vi "Bury.vi"(8 "Error In":errorcluster, 11 "Graves":refnum<vi>[](array[refnum])) -> (0 "Error Out":errorcluster, 3 "Change Made?":bool)   [LabVIEW 2017, in "Toolkit.lvlib"]
doc: "Burys the corpse of legacy code. This removes the grave (Diagram Disable Structure) and leaves behind the Spirit frame, which should be enabled before burying the corpse. Note, the corpse frame will no longer exists and be pernamently deleted."
uses:
  Toolkit.lvlib
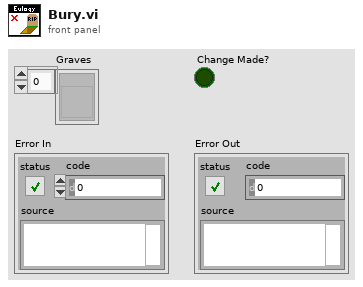
[diagram p1: front panel]
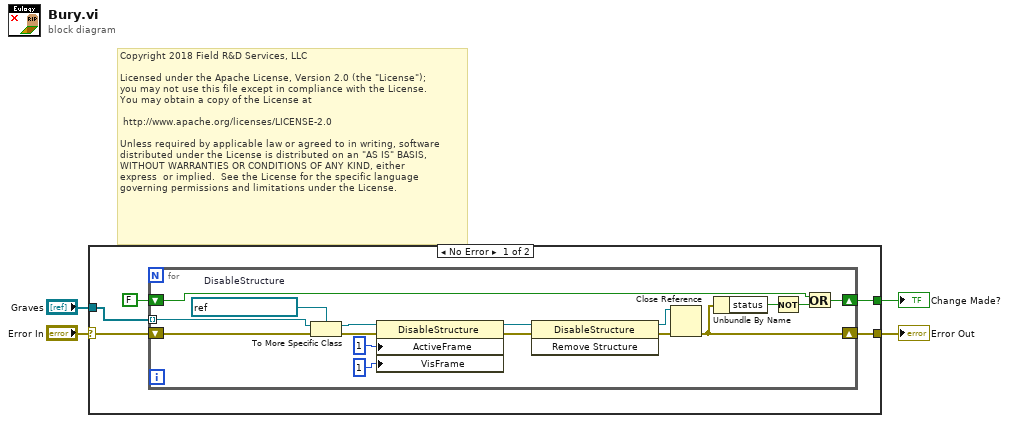
[diagram p0: block diagram]
diagram:
  # "Copyright 2018 Field R&D Services, LLC\n\nLicensed under the Apache License, Version 2.0 (the \"License\");\nyou may not use this file except in compliance with the License.\nYou may obtain a copy of the License at\n\n\thttp://www.apache.org/licenses/LICENSE-2.0\n\nUnless required by applicable law or agreed to in writing, software\ndistributed under the License is distributed on an \"AS IS\" BASIS,\nWITHOUT WARRANTIES OR CONDITIONS OF ANY KIND, either \nexpress  or implied.  See the License for the specific language \ngoverning permissions and limitations under the License."
  n1 = case shown="No Error" "Error In" {
    selector: "Error In" -> [w5 w26]
    tunnel: [w9 w26] -> w4
    tunnel: [w7 _] -> w3
    tunnel: "Graves" -> [w6 _]
    frame No Error {
      n2 = for {
        shift-right: [w12] -> w9
        shift-left: w5 -> [w20]
        tunnel: w6 -> [w21] mode=indexing
        shift-right: [w24] -> w7
        shift-left: FALSE -> [w25]
        w19 = refnum<vi> refnum  # DisableStructure
        n3 = To More Specific Class(target class=w19, reference=w21, error in=w20) -> (specific class reference=w18:refnum<vi>, error out=w17:errorcluster)
        n4 = property class="DisableStructure"(reference=w18, error in=w17, "ActiveFrame"=i16 1 ("Active Frame"), "VisFrame"=u32 1 ("Visible Frame")) -> (reference out=w15:refnum<vi>, error out=w13:errorcluster)
        n5 = invoke class="DisableStructure" method="Remove Structure"(reference=w15, error in=w13) -> (reference out=w22:refnum<vi>, error out=w23:errorcluster)  [unwired: 1 in, 1 out]
        n6 = Close Reference(reference=w22, error in (no error)=w23) -> (error out=w12:errorcluster)
        n7 = Unbundle By Name(w12) -> ("status"=w11:bool)
        n8 = Not(x=w11) -> (.not. x?=w10:bool)
        n9 = Or(x=w25, y=w10) -> (x .or. y?=w24:bool)
      }
    }
    frame Error {
    }
  }
  "Error Out" <- w4
  "Change Made?" <- w3
